vi "Unscaledtoscaled.vi"(2 "Unscaled Data":sgl[](array[numeric]), 3 "Header Information":dbl[](array[numeric])) -> (1 "Array":sgl[](array[numeric]))   [LabVIEW 2015]
doc: "This subVI takes header information and unscaled data and performs a 1D polynomial evaluation to return the scaled data."
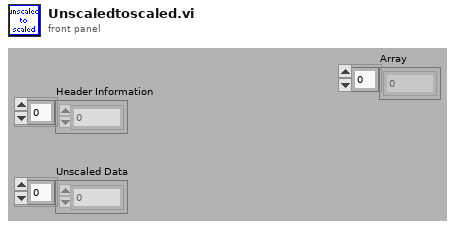
[diagram p1: front panel]
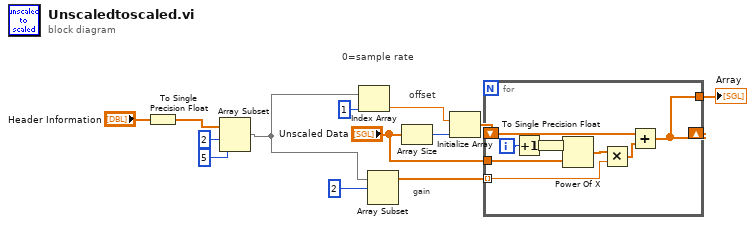
[diagram p0: block diagram]
diagram:
  # "offset"
  # "gain"
  # "0=sample rate"
  n1 = To Single Precision Float(number="Header Information") -> (single precision float=w1:sgl[])
  n2 = Array Subset(array=w1, index=2, length=5) -> (w2:sgl[])
  n3 = Index Array(array=w2, index=1 ("index (row)")) -> (element=w7:sgl)
  n4 = Array Subset(array=w2, index=2) -> (w9:sgl[])  [unwired: 1 in]
  n5 = Array Size(array="Unscaled Data") -> (size(s)=w10:i32)
  n6 = Initialize Array(w7, w10) -> (w11:sgl[])
  n7 = for {
    shift-right: [w15] -> _
    shift-left: w11 -> [w16]
    tunnel: w9 -> [w21] mode=indexing
    tunnel: [w15] -> w6
    tunnel: "Unscaled Data" -> [w20]
    i -> [w22]
    n8 = Increment(x=w22) -> (x+1=w19:i32)
    n9 = To Single Precision Float(number=w19) -> (single precision float=w14:sgl)
    n10 = Power Of X(1:w20, 2:w14) -> (0:w18:sgl[])
    n11 = Multiply(x=w18, y=w21) -> (x*y=w17:sgl[])
    n12 = Add(x=w16, y=w17) -> (x+y=w15:sgl[])
  }
  "Array" <- w6
